vi "DBTester5.vi"() -> ()   [LabVIEW 2015]
uses:
  BERTTA.dll
panel:
  in  "col":i32=3
  out "values":dbl[](array[numeric])
  out "Mettler":dynamicdata(graph)
  in  "Device port":i32=6
  out "Weight":dbl
  out "Weight 2":dbl
  in  "Device port 2":i32=2
  out "rc":i32
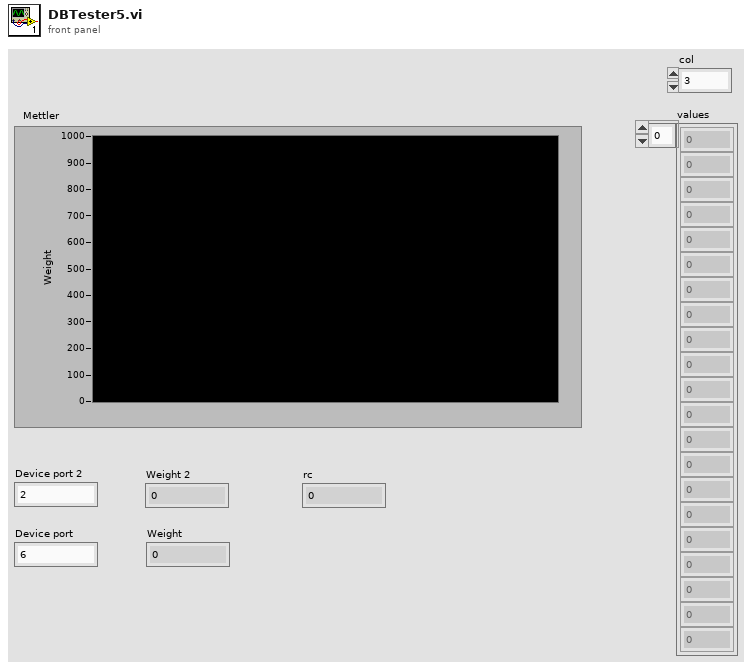
[diagram p1: front panel]
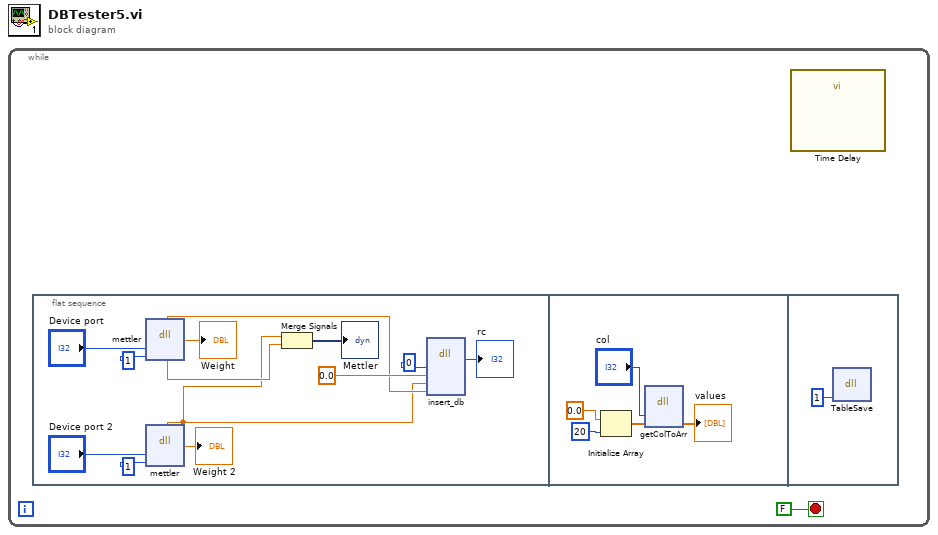
[diagram p0: block diagram]
diagram:
  n1 = while {
    stop <- FALSE stop-if-true
    n2 = flat-sequence {
      frame #0 {
        n3 = dll-call lib="C:/Users/xlaraser/Documents/Visual Studio 2017/Projects/Bertta/BERTTA/Debug/BERTTA.dll" fn="mettler"("port"="Device port", "msg"=1) -> ("return type"=w9:dbl)  [unwired: 5 in, 2 out]
        "Weight" <- w9
        n4 = dll-call lib="C:/Users/xlaraser/Documents/Visual Studio 2017/Projects/Bertta/BERTTA/Debug/BERTTA.dll" fn="mettler"("port"="Device port 2", "msg"=1) -> ("return type"=w8:dbl)  [unwired: 5 in, 2 out]
        "Weight 2" <- w8
        n5 = Merge Signals(w8, w9) -> (→"Mettler":dynamicdata)
        n6 = dll-call lib="C:/Users/xlaraser/Documents/Visual Studio 2017/Projects/Bertta/BERTTA/Debug/BERTTA.dll" fn="insert_db"("heidolph"=0, "lauda"=0.0, "mettler1"=w8, "mettler2"=w9) -> ("return type"=→"rc":i32)  [unwired: 7 in, 2 out]
      }
      frame #1 {
        n7 = Initialize Array(0.0 ("element"), 20 ("dimension size")) -> (w12:dbl[])
        n8 = dll-call lib="C:/Users/xlaraser/Documents/Visual Studio 2017/Projects/Bertta/BERTTA/Debug/BERTTA.dll" fn="getColToArr"("col"="col", "values"=w12) -> ("values"=→"values":dbl[])  [unwired: 5 in, 2 out]
      }
      frame #2 {
        n9 = dll-call lib="C:/Users/xlaraser/Documents/Visual Studio 2017/Projects/Bertta/BERTTA/Debug/BERTTA.dll" fn="TableSave"("exec"=1) -> ()  [unwired: 5 in, 2 out]
      }
    }
    n10 = call "Time Delay"() -> ()  [unwired: 11 in, 1 out]
  }
